vi "设置定时时间.vi"(8 "error in (no error)":errorcluster caption="错误输入（无错误）", 9 "设置时间":u32, 11 "定时器 输入":refnum<class "定时器.lvclass">) -> (0 "error out":errorcluster caption="错误输出", 3 "定时器 输出":refnum<class "定时器.lvclass">)   [LabVIEW 2017, in "定时器.lvclass"]
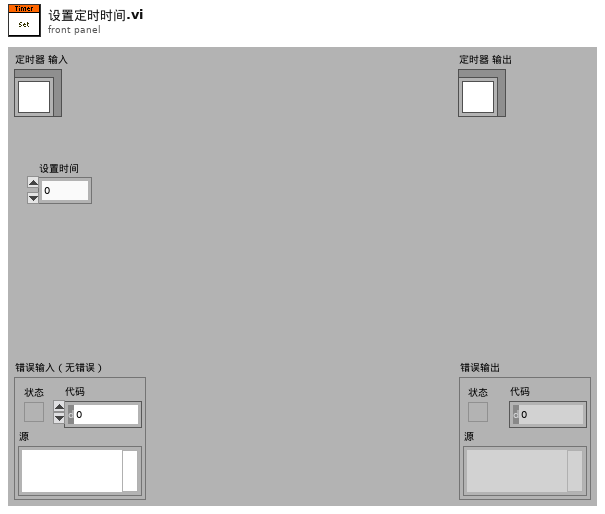
[diagram p1: front panel]
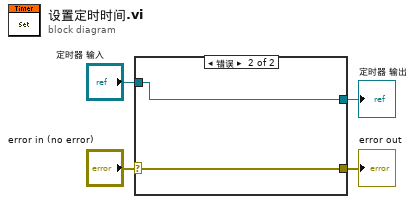
[diagram p0: block diagram]
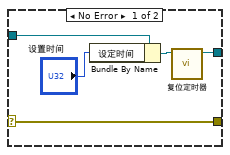
[diagram p2: hidden frame]
diagram:
  n1 = case shown="错误" "error in (no error)" {
    selector: "error in (no error)" -> [w9 w11]
    tunnel: [w9 w11] -> w3
    tunnel: "定时器 输入" -> [w8 w10]
    tunnel: [w5 w10] -> w1
    frame No Error {
      n2 = Bundle By Name(cluster=w8, "设定时间"="设置时间") -> (w6:refnum<class "定时器.lvclass">)
      n3 = call "复位定时器.vi"("定时器 输入"=w6) -> ("定时器 输出"=w5:refnum<class "定时器.lvclass">)  [unwired: 1 in, 9 out]
    }
    frame Error {
    }
  }
  "error out" <- w3
  "定时器 输出" <- w1
